vi "Open OPC UA Connection.vi"(8 "error in (no error)":errorcluster, 10 "OPC UA configuration":refnum<class "OPC UA configuration.lvclass">, 11 "OPC UA runtime in":refnum<class "OPC UA runtime.lvclass">) -> (0 "error out":errorcluster, 3 "OPC UA runtime out":refnum<class "OPC UA runtime.lvclass">)   [LabVIEW 2013, in "OPC UA runtime.lvclass"]
doc: "Opens connection to either an OPC UA Client or Server."
uses:
  OPC UA runtime.lvclass
  configuration/OPC UA configuration.lvclass
  configuration/OPC UA configuration.lvclass/OPC UA configuration.ctl
  OPC UA runtime.lvclass/OPC UA runtime.ctl
  configuration/Read Connection Configuration.vi
  configuration/Read Lines.vi
  <vilib>/NI/Tag Bus Module Framework/channel/TBM channel.lvclass
  <vilib>/opcua/NI OPC UA Server.lvlib
  <vilib>/opcua/NI OPC UA Client.lvlib
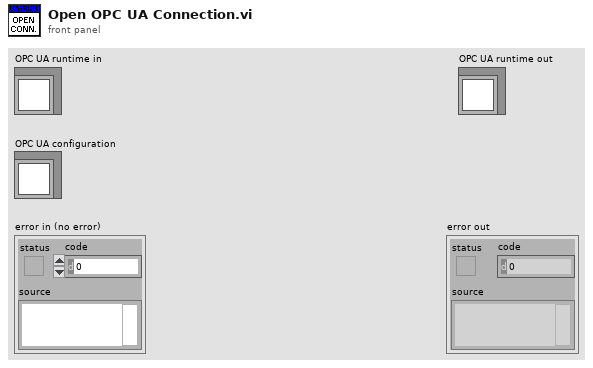
[diagram p1: front panel]
types:
  T1 = typedef "supported security policies.ctl" = cluster{"None":bool, "Sign with Basic128Rsa125":bool, "Sign and Encrypt with Basic128Rsa125":bool, "Sign with Basic256":bool, "Sign and Encrypt with Basic256":bool}
  T2 = cluster{"Client?":bool, "Server Certificates":cluster{"Relative Path?":bool, "Certificate Paths":path[], "Certificate Names":string[]}, "Client Certificates":cluster{"Relative Path?":bool, "Certificate Paths":path[], "Certificate Names":string[]}, "Client Configuration":cluster{"Server Endpoint URL":string, "Security Policy":cluster{"Message Mode":enum16{"None", "Sign", "Sign and Encrypt"}, "Security":enum16{"Basic256", "Basic128Rsa15"}}, "Username/Password":cluster{"Username":string, "Password":string}}, "Server Configuration":cluster{"Server Name":string, "TCP port (49580)":string, "Supported Security Policies":T1}}
  T3 = typedef "OPC UA configuration.lvclass/Line.ctl" = cluster{"channel":refnum<class "TBM channel.lvclass">, "Node Path":string, "OPC UA Data Type":T4}
  T4 = typedef "OPC UA configuration.lvclass/OPC UA Data Type.ctl" = enum16{"Bool", "SByte", "Byte", "Int16", "UInt16", "Int32", "UInt32", "Int64", "UInt64", "Float", "Double", "String", "DateTime", "ByteString", "Bool Array", "SByte Array", "Byte Array", "Int16 Array", "UInt16 Array", "Int32 Array", "UInt32 Array", "Int64 Array", "UInt64 Array", "Float Array", "Double Array", "String Array", "DateTime Array", "ByteString Array"}
  T5 = cluster{"Relative Path?":bool, "Certificate Paths":path[], "Certificate Names":string[]}
  T6 = cluster{"Message Mode":enum16{"None", "Sign", "Sign and Encrypt"}, "Security":enum16{"Basic256", "Basic128Rsa15"}}
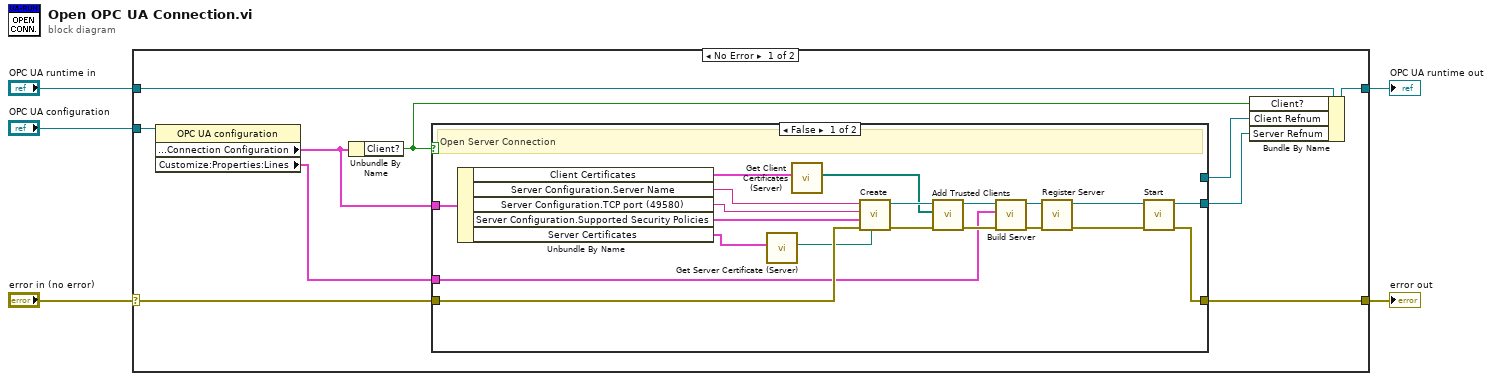
[diagram p0: block diagram]
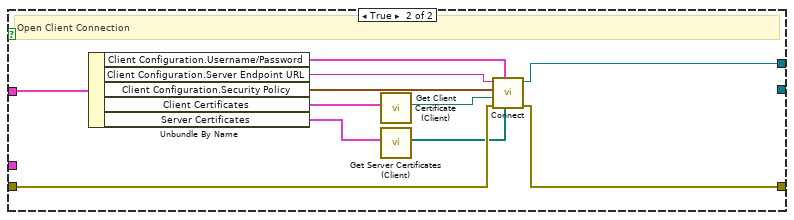
[diagram p2: hidden frame]
diagram:
  n1 = case shown="No Error" "error in (no error)" {
    selector: "error in (no error)" -> [w12 w48]
    tunnel: [w10 w48] -> w4
    tunnel: [w14 w47] -> w2
    tunnel: "OPC UA runtime in" -> [w15 w47]
    tunnel: "OPC UA configuration" -> [w7 _]
    frame No Error {
      n2 = property class="OPC UA configuration"(reference=w7) -> ("Customize:Properties:Connection Configuration"=w8:T2, "Customize:Properties:Lines"=w6:T3[])  [unwired: 1 in, 2 out]
      n3 = Unbundle By Name(w8) -> ("Client?"=w13:bool)
      n4 = case shown="False" w13 {
        tunnel: w8 -> [w35 w43]
        tunnel: w12 -> [w34 w46]
        tunnel: [w23 _] -> w11
        tunnel: [w24 w45] -> w10
        tunnel: [_ w44] -> w9
        tunnel: w6 -> [w16 _]
        frame False {
          # "Open Server Connection"
          n5 = Unbundle By Name(w35) -> ("Client Certificates"=w26:T5, "Server Configuration.Server Name"=w31:string, "Server Configuration.TCP port (49580)"=w32:string, "Server Configuration.Supported Security Policies"=w33:T1, "Server Certificates"=w30:T5)
          n6 = call "Get Server Certificate (Server).vi"("Server Certificates"=w30) -> ("server certificate file"=w29:path)  [unwired: 10 in]
          n7 = call "Get Client Certificates (Server).vi"("Client Certificates"=w26) -> ("trusted client certificates"=w25:path[])  [unwired: 10 in]
          n8 = call <vilib>:"Create.vi"("server certificate file"=w29, "error in (no error)"=w34, "supported security policies (None)"=w33, "TCP port (49580)"=w32, "OPC UA server name"=w31) -> ("error out"=w28:errorcluster, "OPC UA server refnum out"=w27:refnum<k21>)  [unwired: 4 in, 1 out]
          n9 = call <vilib>:"Add Trusted Clients.vi"("error in (no error)"=w28, "trusted client certificates"=w25, "OPC UA server refnum in"=w27) -> ("error out"=w21:errorcluster, "OPC UA server refnum out"=w22:refnum<k21>)  [unwired: 7 in]
          n10 = call "Build Server.vi"("Error In"=w21, "Lines"=w16, "OPC UA server refnum in"=w22) -> ("Error Out"=w19:errorcluster, "OPC UA server refnum out"=w20:refnum<k21>)  [unwired: 7 in]
          n11 = call <vilib>:"Register Server.vi"("error in (no error)"=w19, "OPC UA server refnum in"=w20) -> ("error out"=w18:errorcluster, "OPC UA server refnum out"=w17:refnum<k21>)  [unwired: 8 in]
          n12 = call <vilib>:"Start.vi"("error in (no error)"=w18, "OPC UA server refnum in"=w17) -> ("error out"=w24:errorcluster, "OPC UA server refnum out"=w23:refnum<k21>)  [unwired: 8 in]
        }
        frame True {
          # "Open Client Connection"
          n13 = Unbundle By Name(w43) -> ("Client Configuration.Username/Password"=w42:cluster{"Username":string, "Password":string}, "Client Configuration.Server Endpoint URL"=w41:string, "Client Configuration.Security Policy"=w40:T6, "Client Certificates"=w39:T5, "Server Certificates"=w37:T5)
          n14 = call "Get Client Certificate (Client).vi"("Client Certificates"=w39) -> ("client certificate file"=w38:path)  [unwired: 10 in]
          n15 = call "Get Server Certificates (Client).vi"("Server Certificates"=w37) -> ("trusted server certificates"=w36:path[])  [unwired: 10 in]
          n16 = call <vilib>:"Connect.vi"("trusted server certificates"=w36, "username/password"=w42, "error in (no error)"=w46, "client certificate file"=w38, "security policy"=w40, "server endpoint URL"=w41) -> ("error out"=w45:errorcluster, "OPC UA client refnum out"=w44:refnum<k21>)  [unwired: 3 in, 1 out]
        }
      }
      n17 = Bundle By Name(cluster=w15, "Client?"=w13, "Client Refnum"=w9, "Server Refnum"=w11) -> (w14:refnum<class "OPC UA runtime.lvclass">)
    }
    frame Error {
    }
  }
  "error out" <- w4
  "OPC UA runtime out" <- w2
